vi "_PC_NS_Signal_Process.vi"(4 "Stop":refnum<vi>, 5 "SysMsg":refnum<vi>, 6 "Maximum Reader":i32=20, 7 "Conn_Bool":refnum<data-value>, 8 "error in (no error)":errorcluster, 9 "# signal in NS ref":refnum<vi>, 11 "Sig Queue":refnum<queue>) -> (0 "error out":errorcluster)   [LabVIEW 2018]
uses:
  <vilib>/Platform/TimedLoop/XDataNode/timing_clust.ctl
  <vilib>/Platform/TimedLoop/XDataNode/nitl_modes.ctl
  <vilib>/Platform/TimedLoop/XDataNode/wakeup.ctl
  <vilib>/Platform/TimedLoop/XDataNode/XDataNode.xnode
  PC_NS_Signal.lvclass
  <vilib>/Platform/TimedLoop/XDataNode/XDNodeRunTimeDep.lvlib
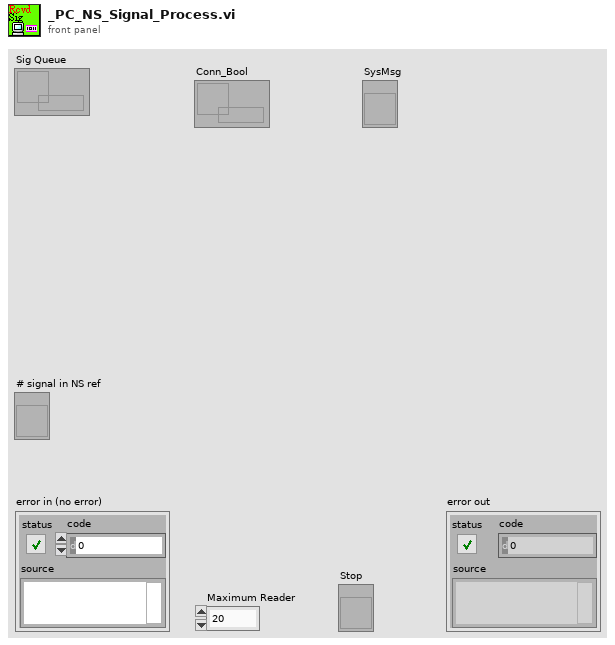
[diagram p1: front panel]
types:
  T1 = typedef "XDNodeRunTimeDep.lvlib/timing_clust.ctl" = cluster{"Expected End [f-1]":u64, "Actual End [f-1]":u64, "Finished Late? [f-1]":bool, "Expected End [i-1]":u64, "Actual End [i-1]":u64, "Finished Late? [i-1]":bool, "Expected Start [i]":u64, "Actual Start [i]":u64, "Expected Start [f]":u64, "Actual Start [f]":u64, "Source Name":string, "Structure Name":string, "Period":i64, "Deadline":i64, "Offset":i64, "Start":i64, "Priority":i32, "Timeout":i32, "Mode":T2, "Wakeup Reason":T3, "Error":errorcluster, "Source Type":string, "Secondary Source Type":string, "Global End Time":u64, "Global Start Time":u64, "Frame Duration":u64, "Iteration Duration":u64, "Assigned CPU":i32, "I/O Scan Engine Mode":u32}
  T2 = typedef "XDNodeRunTimeDep.lvlib/nitl_modes.ctl" = enum32{"No Change", "Process missed periods, maintain original phase", "Discard missed periods, maintain original phase", "Process missed periods, ignore original phase", "Discard missed periods, ignore original phase"}
  T3 = typedef "XDNodeRunTimeDep.lvlib/wakeup.ctl" = enum32{"Normal", "Aborted", "Asynchronous wakeup", "Timing source error", "Timed loop error", "Timeout"}
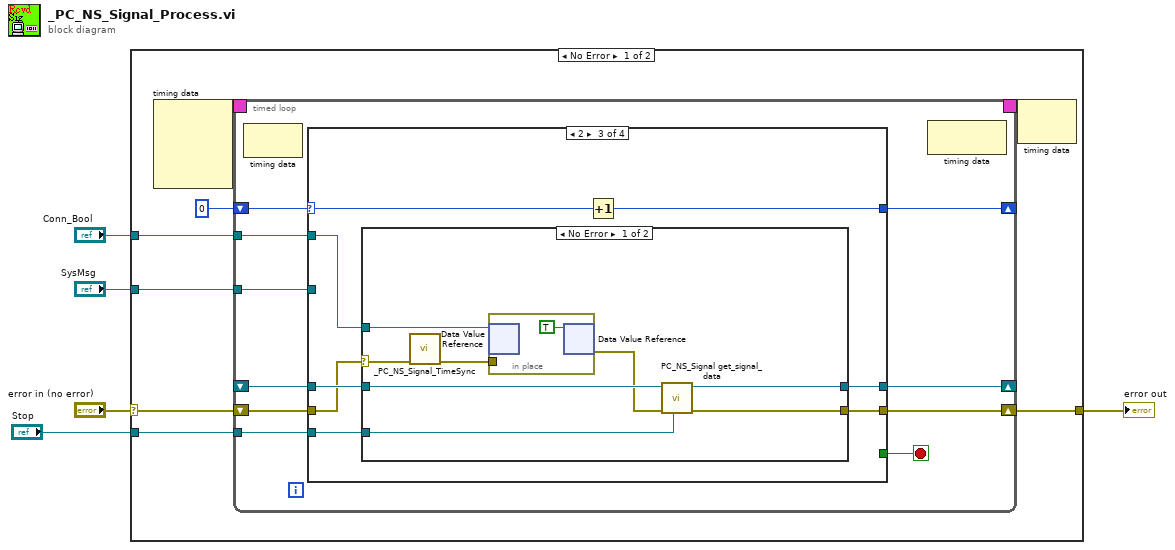
[diagram p0: block diagram]
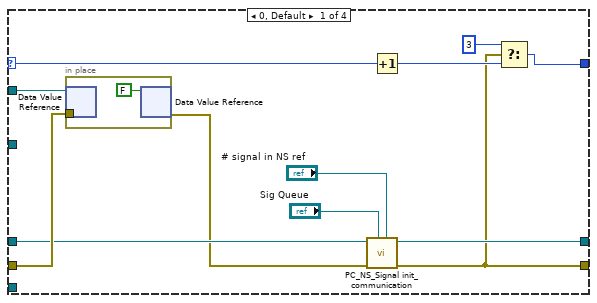
[diagram p2: hidden frame]
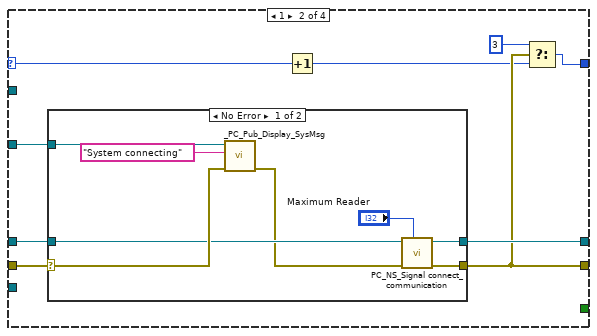
[diagram p3: hidden frame]
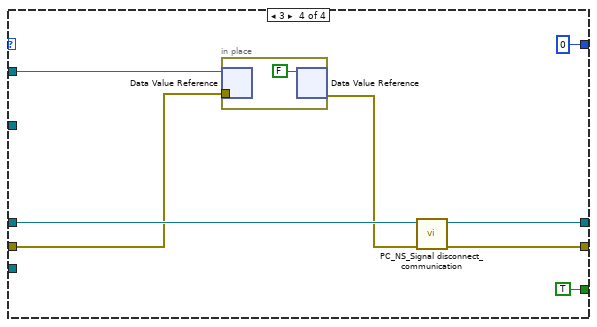
[diagram p6: hidden frame]
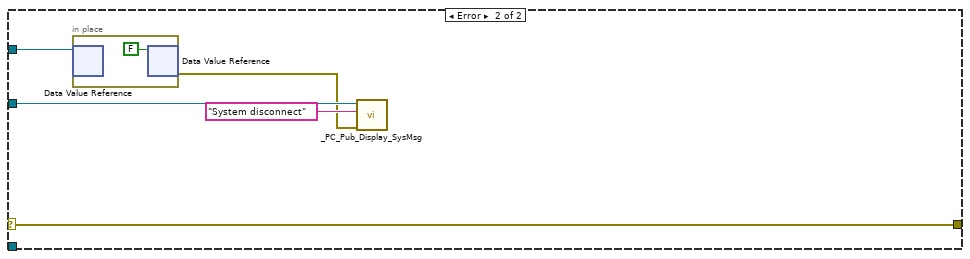
[diagram p7: hidden frame]
diagram:
  n1 = case shown="No Error" "error in (no error)" {
    selector: "error in (no error)" -> [w12 w89]
    tunnel: "Conn_Bool" -> [w11 w91]
    tunnel: "SysMsg" -> [w10 w90]
    tunnel: [w9 w89] -> w2
    tunnel: "Stop" -> [w6 _]
    frame No Error {
      n2 = node-c288() -> (w8:T1)  [unwired: 4 in]
      n3 = timed-loop {
        shift-right: [w16] -> w9
        shift-left: w12 -> [w23]
        shift-right: [w15] -> _
        shift-left: u8 0 -> [w22]
        tunnel: w10 -> [w20]
        tunnel: w11 -> [w19]
        shift-right: [w18] -> _
        shift-left: _ -> [w17]
        timing: w8 -> [_]
        timing-out: [_] -> w7
        tunnel: w6 -> [w14]
        stop <- w21 stop-if-true
        n4 = node-c288() -> ()  [unwired: 1 in, 1 out]
        n5 = case shown="2" w22 {
          selector: w22 -> [w37 w47 w64 _]
          tunnel: w23 -> [w32 w45 w60 w79]
          tunnel: [w27 w42 w65 w81] -> w16
          tunnel: [_ _ _ TRUE] -> w21
          tunnel: w20 -> [_ w46 _ _]
          tunnel: w19 -> [w36 _ w59 w84]
          tunnel: [w33 w43 w62 w82] -> w18
          tunnel: w17 -> [w31 w44 w63 w83]
          tunnel: [w26 w40 w61 u8 0] -> w15
          tunnel: w14 -> [_ _ w58 _]
          frame 0, Default {
            n6 = in-place {
              in-place-border: w32 -> [_]
              n7 = in-place-dvr #1(w36) -> ()  [unwired: 2 out]
              n8 = in-place-dvr #1(FALSE ("data value")) -> (w30:errorcluster)  [unwired: 1 out]
            }
            n9 = call "PC_NS_Signal init_communication.vi"("# signal in NS ref"="# signal in NS ref", "sig queue"="Sig Queue", "error in (no error)"=w30, "PC_NS_Signal in"=w31) -> ("error out"=w27:errorcluster, "PC_NS_Signal out"=w33:refnum<class "PC_NS_Signal.lvclass">)  [unwired: 6 in]
            n10 = Increment(x=w37) -> (x+1=w29:u8)
            n11 = Select(t=u8 3, s=w27, f=w29) -> (s? t:f=w26:u8)
          }
          frame 1 {
            n12 = case shown="No Error" w45 {
              selector: w45 -> [w53 w57]
              tunnel: [w50 w56] -> w43
              tunnel: w46 -> [w54 _]
              tunnel: [w48 w57] -> w42
              tunnel: w44 -> [w51 w56]
              frame No Error {
                n13 = call "_PC_Pub_Display_SysMsg.vi"("error in (no error)"=w53, "Msg String"="System connecting" ("Msg in"), "SysMsg Ref In"=w54) -> ("error out"=w49:errorcluster)  [unwired: 7 in, 1 out]
                n14 = call "PC_NS_Signal connect_communication.vi"("Maximum Reader"="Maximum Reader", "error in (no error)"=w49, "PC_NS_Signal in"=w51) -> ("error out"=w48:errorcluster, "PC_NS_Signal out"=w50:refnum<class "PC_NS_Signal.lvclass">)  [unwired: 7 in]
              }
              frame Error {
              }
            }
            n15 = Increment(x=w47) -> (x+1=w41:u8)
            n16 = Select(t=u8 3, s=w42, f=w41) -> (s? t:f=w40:u8)
          }
          frame 2 {
            n17 = case shown="No Error" w60 {
              selector: w60 -> [w68 w76]
              tunnel: [w71 w76] -> w65
              tunnel: [w72 w75] -> w62
              tunnel: w63 -> [w73 w75]
              tunnel: w59 -> [w70 _]
              tunnel: w58 -> [w66 _]
              frame No Error {
                n18 = call "_PC_NS_Signal_TimeSync.vi"("error in (no error)"=w68) -> ("error out"=w67:errorcluster)  [unwired: 10 in]
                n19 = in-place {
                  in-place-border: w67 -> [_]
                  n20 = in-place-dvr #2(w70) -> ()  [unwired: 2 out]
                  n21 = in-place-dvr #2(TRUE ("data value")) -> (w69:errorcluster)  [unwired: 1 out]
                }
                n22 = call "PC_NS_Signal get_signal_data.vi"("Stop"=w66, "error in (no error)"=w69, "PC_NS_Signal in"=w73) -> ("error out"=w71:errorcluster, "PC_NS_Signal out"=w72:refnum<class "PC_NS_Signal.lvclass">)  [unwired: 7 in]
              }
              frame Error {
              }
            }
            n23 = Increment(x=w64) -> (x+1=w61:u8)
          }
          frame 3 {
            n24 = in-place {
              in-place-border: w79 -> [_]
              n25 = in-place-dvr #3(w84) -> ()  [unwired: 2 out]
              n26 = in-place-dvr #3(FALSE ("data value")) -> (w77:errorcluster)  [unwired: 1 out]
            }
            n27 = call "PC_NS_Signal disconnect_communication.vi"("error in (no error)"=w77, "PC_NS_Signal in"=w83) -> ("error out"=w81:errorcluster, "PC_NS_Signal out"=w82:refnum<class "PC_NS_Signal.lvclass">)  [unwired: 8 in]
          }
        }
        n28 = node-c288() -> ()  [unwired: 1 in, 1 out]
      }
      n29 = node-c288(w7) -> ()  [unwired: 1 out]
    }
    frame Error {
      n30 = in-place {
        n31 = in-place-dvr #4(w91) -> ()  [unwired: 2 out]
        n32 = in-place-dvr #4(FALSE ("data value")) -> (w88:errorcluster)  [unwired: 1 out]
      }
      n33 = call "_PC_Pub_Display_SysMsg.vi"("error in (no error)"=w88, "Msg String"="System disconnect" ("Msg in"), "SysMsg Ref In"=w90) -> ()  [unwired: 7 in, 2 out]
    }
  }
  "error out" <- w2
